vi "Aero_Tunnel_Server_Global.vi"() -> ()   [LabVIEW 2010]
panel:
  out "SmAD Data":dbl[](array[numeric]) format="%.2f"
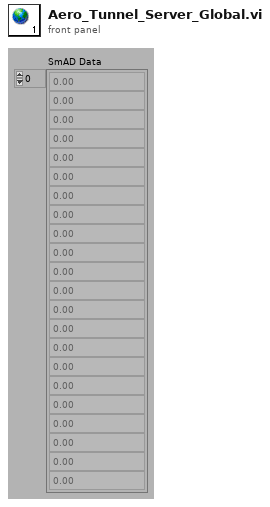
[diagram p1: front panel]
diagram:
